vi "AvarageSamples.vi"(11 "samples":dbl[](array[numeric])) -> (3 "Avg":dbl)   [LabVIEW 2021]
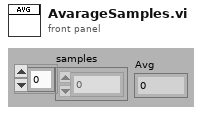
[diagram p1: front panel]
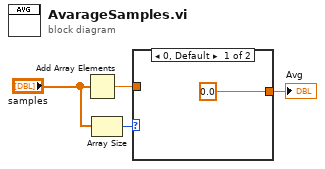
[diagram p0: block diagram]
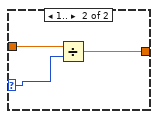
[diagram p2: hidden frame]
diagram:
  n1 = Add Array Elements(numeric array="samples") -> (sum=w2:dbl)
  n2 = Array Size(array="samples") -> (size(s)=w4:i32)
  n3 = case shown="0, Default" w4 {
    selector: w4 -> [_ w7]
    tunnel: w2 -> [_ w8]
    tunnel: [0.0 w6] -> w1
    frame 0, Default {
    }
    frame 1.. {
      n4 = Divide(x=w8, y=w7) -> (x/y=w6:dbl)
    }
  }
  "Avg" <- w1
